vi "TSA_AR_Modeling_array.vi"(9 "AR order":i32=4, 10 "method":u16(ring) items=["Forward-Backward", "Least-Squares", "Yule-Walker", "Burg-Lattice", "Geometric-Lattice"], 11 "Xt":dbl[](array[numeric]) format="%.2f") -> (0 "error":i32, 1 "noise":dbl[](array[numeric]) format="%.10f", 2 "sita^2":dbl, 3 "AR coefficients":dbl[](array[numeric]))   [LabVIEW 2014, in "NI_AALPro.lvlib"]
doc: "Estimates the autoregressive (AR) model of an input univariate or multivariate (vector) time series according to the method you specify."
uses:
  NI_AALPro.lvlib
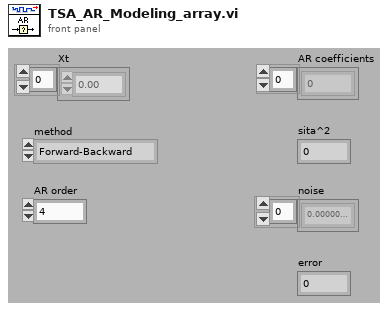
[diagram p1: front panel]
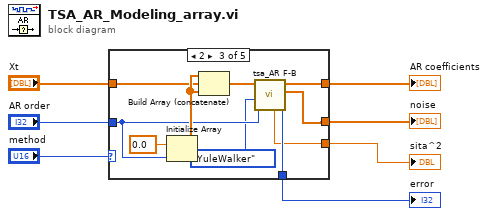
[diagram p0: block diagram]
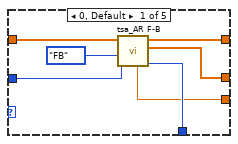
[diagram p2: hidden frame]
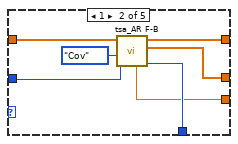
[diagram p3: hidden frame]
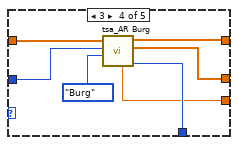
[diagram p4: hidden frame]
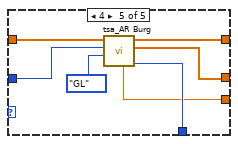
[diagram p5: hidden frame]
diagram:
  n1 = case shown="2" "method" {
    tunnel: "Xt" -> [w14 w21 w29 w38 w44]
    tunnel: "AR order" -> [w13 w19 w26 w35 w42]
    tunnel: [w11 w20 w27 w37 w43] -> w6
    tunnel: [w10 w18 w25 w36 w41] -> w1
    tunnel: [w9 w17 w24 w33 w40] -> w5
    tunnel: [w8 w15 w23 w32 w39] -> w2
    frame 0, Default {
      n2 = call "tsa_AR F-B.vi"("method"=enum16{"FB", "Cov", "YuleWalker"}."FB", "AR order"=w13, "response signal"=w14) -> ("error"=w10:i32, "noise"=w9:dbl[], "AR coefficents"=w11:dbl[], "sita^2"=w8:dbl)  [unwired: 4 in, 1 out]
    }
    frame 1 {
      n3 = call "tsa_AR F-B.vi"("method"=enum16{"FB", "Cov", "YuleWalker"}."Cov", "AR order"=w19, "response signal"=w21) -> ("error"=w18:i32, "noise"=w17:dbl[], "AR coefficents"=w20:dbl[], "sita^2"=w15:dbl)  [unwired: 4 in, 1 out]
    }
    frame 2 {
      n4 = Initialize Array(0.0 ("element"), w26) -> (w30:dbl[])
      n5 = Build Array (concatenate)(w30, w29, w30) -> (w28:dbl[])
      n6 = call "tsa_AR F-B.vi"("method"=enum16{"FB", "Cov", "YuleWalker"}."YuleWalker", "AR order"=w26, "response signal"=w28) -> ("error"=w25:i32, "noise"=w24:dbl[], "AR coefficents"=w27:dbl[], "sita^2"=w23:dbl)  [unwired: 4 in, 1 out]
    }
    frame 3 {
      n7 = call "tsa_AR Burg.vi"("method"=enum16{"Burg", "GL"}."Burg", "AR order"=w35, "response signal"=w38) -> ("error"=w36:i32, "noise"=w33:dbl[], "AR coefficents"=w37:dbl[], "sita^2"=w32:dbl)  [unwired: 4 in, 1 out]
    }
    frame 4 {
      n8 = call "tsa_AR Burg.vi"("method"=enum16{"Burg", "GL"}."GL", "AR order"=w42, "response signal"=w44) -> ("error"=w41:i32, "noise"=w40:dbl[], "AR coefficents"=w43:dbl[], "sita^2"=w39:dbl)  [unwired: 4 in, 1 out]
    }
  }
  "AR coefficients" <- w6
  "noise" <- w5
  "sita^2" <- w2
  "error" <- w1
